vi "Wait on Connection.vi"(8 "error in (no error)":errorcluster, 10 "Timeout (25000 ms)":i32=25000, 11 "TCP Server in":refnum<class "TCP Server.lvclass">) -> (0 "error out":errorcluster, 2 "Connection":refnum<class "IConnection.lvclass">, 3 "TCP Server out":refnum<class "TCP Server.lvclass">)   [LabVIEW 2017, in "TCP Interface.lvlib" / "TCP Server.lvclass"]
uses:
  <vilib>/gpm_packages/@cs/Network-sink/Source/TCP Interface/TCP Server/TCP Server.lvclass
  <vilib>/gpm_packages/@cs/Network-sink/Source/Network Interface/IConnection/IConnection.lvclass
  <vilib>/gpm_packages/@cs/Network-sink/Source/TCP Interface/TCP Server/TCP Server.lvclass/TCP Server.ctl
  <vilib>/gpm_packages/@cs/Network-sink/Source/TCP Interface/TCP Connection/TCP Connection.lvclass
  C:/Program Files/National Instruments/LabVIEW 2017/vi.lib/gpm_packages/@cs/Network-sink/Source/Network Interface/IConnection/IConnection.lvclass
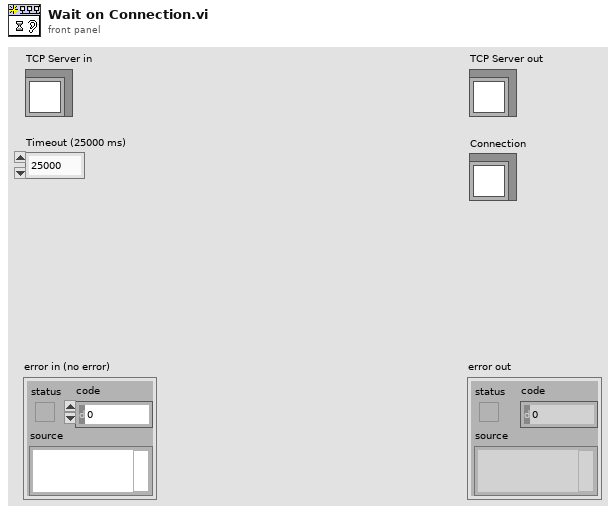
[diagram p1: front panel]
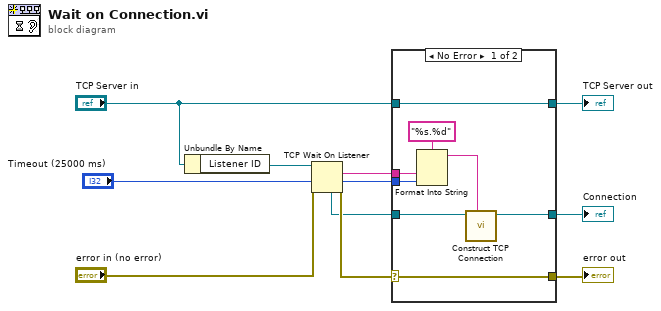
[diagram p0: block diagram]
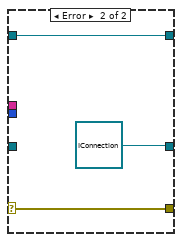
[diagram p2: hidden frame]
diagram:
  n1 = Unbundle By Name("TCP Server in") -> ("Listener ID"=w9:refnum<k5>)
  n2 = TCP Wait On Listener(8:"error in (no error)", 9:"Timeout (25000 ms)", 11:w9) -> (0:w6:errorcluster, 1:w1:u16, 2:w2:string, 4:w5:refnum<k5>)  [unwired: 1 in, 1 out]
  n3 = case shown="No Error" w6 {
    selector: w6 -> [w16 w21]
    tunnel: "TCP Server in" -> [w19 w22]
    tunnel: [w19 w22] -> w11
    tunnel: w5 -> [w18 _]
    tunnel: [w16 w21] -> w4
    tunnel: [w17 refnum<class "IConnection.lvclass"> refnum ("Connection")] -> w3
    tunnel: w2 -> [w15 _]
    tunnel: w1 -> [w14 _]
    frame No Error {
      n4 = Format Into String(format string="%s.%d", w15, w14) -> (resulting string=w12:string)  [unwired: 2 in, 1 out]
      n5 = call <vilib>:"Construct TCP Connection.vi"("ID"=w12, "ConnectionRef"=w18) -> ("TCP Connection out"=w17:refnum<class "TCP Connection.lvclass">)  [unwired: 9 in]
    }
    frame Error {
    }
  }
  "error out" <- w4
  "TCP Server out" <- w11
  "Connection" <- w3
